vi "Set Pulse Length.vi"(7 "Ref Pulse Range":refnum<vi>, 8 "error in":errorcluster, 9 "Head Channel":i16, 10 "Pulsar Handle":i16, 11 "OphirFastX (in)":refnum<k7>) -> (0 "error out":errorcluster, 3 "OphirFastX (out)":refnum<k7>)   [LabVIEW 2009]
panel:
  # "Guillaume Plateau - yguig2@yahoo.fr"
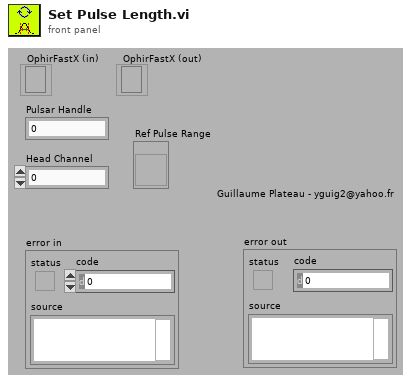
[diagram p1: front panel]
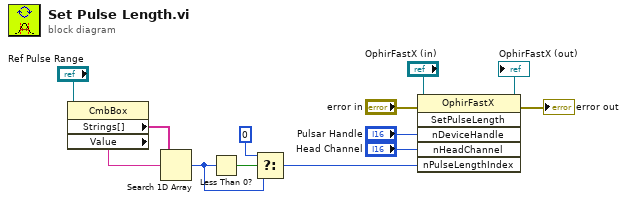
[diagram p0: block diagram]
diagram:
  n1 = property class="CmbBox"(reference="Ref Pulse Range") -> ("Strings[]"=w6:string[], "Value"=w5:string)  [unwired: 1 in, 2 out]
  n2 = Search 1D Array(1D array=w6, element=w5) -> (index of element=w2:i32)  [unwired: 1 in]
  n3 = Less Than 0?(x=w2) -> (x < 0?=w4:bool)
  n4 = Select(t=i16 0 ("nRangeIndex"), s=w4, f=w2) -> (s? t:f=w1:i32)
  n5 = invoke class="OphirFastX" method="SetPulseLength"(reference="OphirFastX (in)", error in="error in", "nDeviceHandle"="Pulsar Handle", "nHeadChannel"="Head Channel", "nPulseLengthIndex"=w1) -> (reference out=→"OphirFastX (out)":refnum<k7>, error out=→"error out":errorcluster)  [unwired: 1 in, 4 out]
